vi "AlliGator Source Image Display Mouse Down-Up Event Monitoring.vi"(0 "Source Image Display Event Registration":refnum<event-registration>, 5 "Source Image Display Refnum":T1, 11 "Error In":errorcluster, 12 "Look for Mouse Down(T)/Up(F)":bool) -> (4 "Source Image Display Event Registration":refnum<event-registration>, 15 "Error Out":errorcluster)   [LabVIEW 2021, in "AlliGator GUI.lvlib"]
doc: "Updates registered events associated with the Source Image upon mouse click."
uses:
  Image/Image Control Refnum.ctl
  AlliGator GUI.lvlib
  Image/Image.lvlib
panel:
  # "see the AlliGator License on the block diagram (Ctrl+E or Window:Show Block Diagram)"
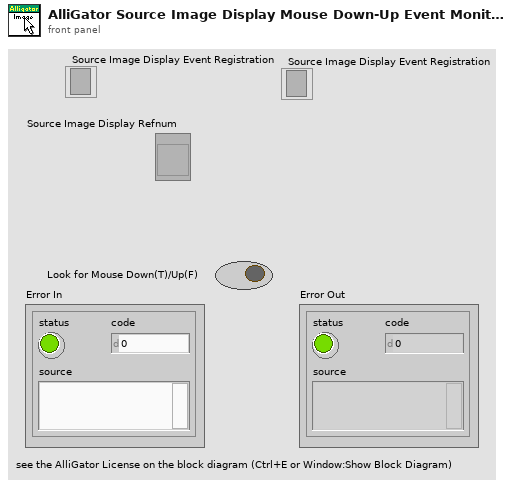
[diagram p1: front panel]
types:
  T1 = typedef "Image.lvlib/Image Control Refnum.ctl" = refnum<vi>
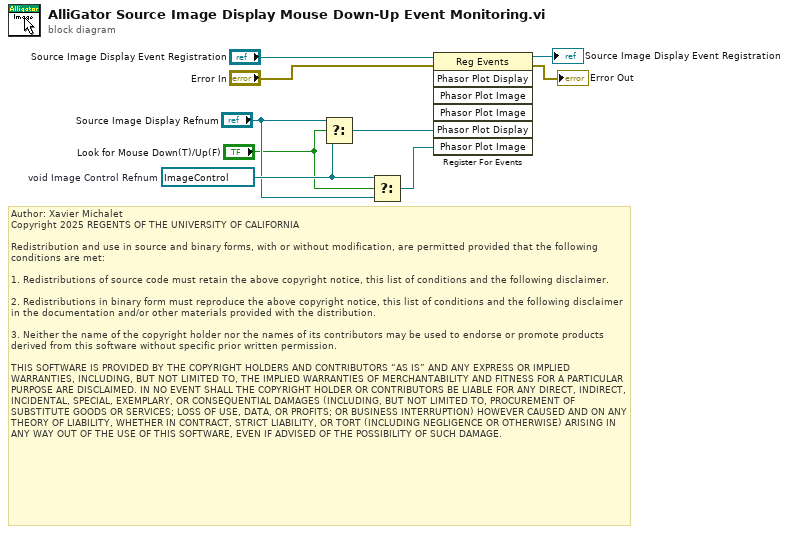
[diagram p0: block diagram]
diagram:
  w9 = refnum<vi> refnum  # void Image Control Refnum
  # "Author: Xavier Michalet\nCopyright 2025 REGENTS OF THE UNIVERSITY OF CALIFORNIA\n\nRedistribution and use in source and binary forms, with or without modification, are permitted provided that the following conditions are met:\n\n1. Redistributions of source code must retain the above copyright notice, this list of conditions and the following disclaimer.\n\n2. Redistributions in binary form must reproduce the above copyright notice, this list of conditions and the following disclaimer in the documentation and/or other materials provided with the distribution.\n\n3. Neither the name of the copyright holder nor the names of its contributors may be used to endorse or promote products derived from this software without specific prior written permission.\n\nTHIS SOFTWARE IS PROVIDED BY THE COPYRIGHT HOLDERS AND CONTRIBUTORS “AS IS” AND ANY EXPRESS OR IMPLIED WARRANTIES, INCLUDING, BUT NOT LIMITED TO, THE IMPLIED WARRANTIES OF MERCHANTABILITY AND FITNESS FOR A PARTICULAR PURPOSE ARE DISCLAIMED. IN NO EVENT SHALL THE COPYRIGHT HOLDER OR CONTRIBUTORS BE LIABLE FOR ANY DIRECT, INDIRECT, INCIDENTAL, SPECIAL, EXEMPLARY, OR CONSEQUENTIAL DAMAGES (INCLUDING, BUT NOT LIMITED TO, PROCUREMENT OF SUBSTITUTE GOODS OR SERVICES; LOSS OF USE, DATA, OR PROFITS; OR BUSINESS INTERRUPTION) HOWEVER CAUSED AND ON ANY THEORY OF LIABILITY, WHETHER IN CONTRACT, STRICT LIABILITY, OR TORT (INCLUDING NEGLIGENCE OR OTHERWISE) ARISING IN ANY WAY OUT OF THE USE OF THIS SOFTWARE, EVEN IF ADVISED OF THE POSSIBILITY OF SUCH DAMAGE."
  n1 = Select(t="Source Image Display Refnum", s="Look for Mouse Down(T)/Up(F)", f=w9) -> (s? t:f=w4:T1)
  n2 = Select(t=w9, s="Look for Mouse Down(T)/Up(F)", f="Source Image Display Refnum") -> (s? t:f=w3:T1)
  n3 = register-events(reference="Source Image Display Event Registration", error in="Error In", w4, w3) -> (reference out=→"Source Image Display Event Registration":refnum<event-registration>, error out=→"Error Out":errorcluster)  [unwired: 3 in]
